vi "ResetSMU.vi"(7 "SMU":T1, 8 "Error In":errorcluster, 11 "Keithley 2602 In":refnum<visa-resource-name>) -> (0 "Error Out":errorcluster, 3 "Keithley 2602 Out":refnum<visa-resource-name>)   [LabVIEW 2012, in "Keithley-2602.lvlib"]
uses:
  Keithley-2602.lvlib
  Controls/SMU.ctl
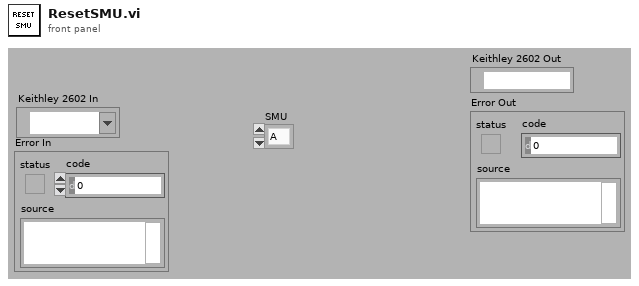
[diagram p1: front panel]
types:
  T1 = typedef "Keithley-2602.lvlib/SMU.ctl" = enum16{"A", "B"}
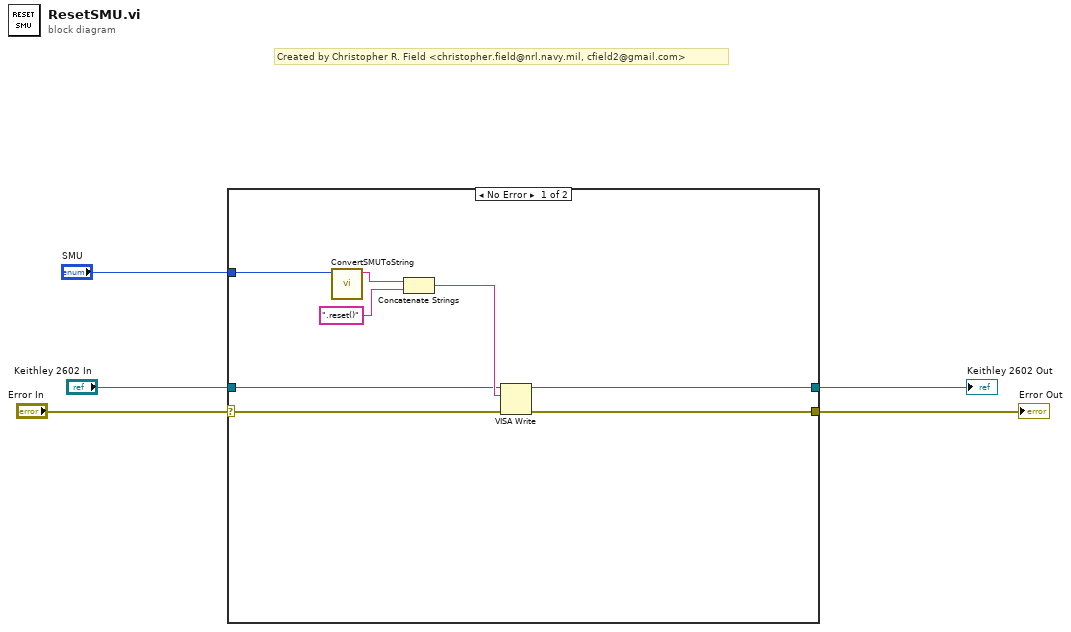
[diagram p0: block diagram]
diagram:
  # "Created by Christopher R. Field <christopher.field@nrl.navy.mil, cfield2@gmail.com>"
  n1 = case shown="No Error" "Error In" {
    selector: "Error In" -> [w6 w14]
    tunnel: "Keithley 2602 In" -> [w10 w15]
    tunnel: [w9 w15] -> w4
    tunnel: [w8 w14] -> w3
    tunnel: "SMU" -> [w7 _]
    frame No Error {
      n2 = call "ConvertSMUToString.vi"("SMU"=w7) -> ("Channel"=w13:string)  [unwired: 10 in]
      n3 = Concatenate Strings(w13, ".reset()") -> (w11:string)
      n4 = VISA Write(VISA resource name=w10, write buffer=w11, error in (no error)=w6) -> (VISA resource name out=w9:refnum<visa-resource-name>, error out=w8:errorcluster)  [unwired: 1 out]
    }
    frame Error {
    }
  }
  "Keithley 2602 Out" <- w4
  "Error Out" <- w3
